vi "FPGA PID control.vi"(4 "PID output channel":T1, 5 "output ranges":T9={"output high (Inf)"=inf, "output low (-Inf)"=-inf}, 6 "reset pid":T7, 7 "PID gains":T8 {"filter coefficient" min=0 max=1; "proportional gain" step=0.125}, 8 "PID input channel":T1, 9 "setpoint":T5, 10 "set output":T3=[0.0, 0.0, 0.0, 0.0], 11 "inputs":T4=[0.0, 0.0, 0.0, 0.0]) -> (1 "PID status":T6, 2 "to AO channels":T2, 3 "actual outputs":sgl[](array[numeric]))   [LabVIEW 2016]
uses:
  Type Def Ctrls/FPGA ctrls/PID output selection.ctl
  <vilib>/rvi/Analysis/control/PID/Typedef/niFpgaPID_OutputRange.ctl
  <vilib>/rvi/Analysis/control/PID/Typedef/niFpgaPID_PIDGains.ctl
  Type Def Ctrls/FPGA ctrls/Reset PID.ctl
  Type Def Ctrls/FPGA ctrls/PID status.ctl
  Type Def Ctrls/FPGA ctrls/Manual Setpoint.ctl
  Type Def Ctrls/FPGA ctrls/Input Channels.ctl
  Type Def Ctrls/FPGA ctrls/Output Channels.ctl
  Type Def Ctrls/FPGA ctrls/AO channel cluster.ctl
  <vilib>/rvi/Emulation/niFpgaSctlEmulationGetInTimedLoop.vi
  <vilib>/rvi/Emulation/niFpgaProcessEmulError.vi
  <vilib>/rvi/Analysis/control/PID/SubVIs/niFpgaPID_PIDWrapper.vi
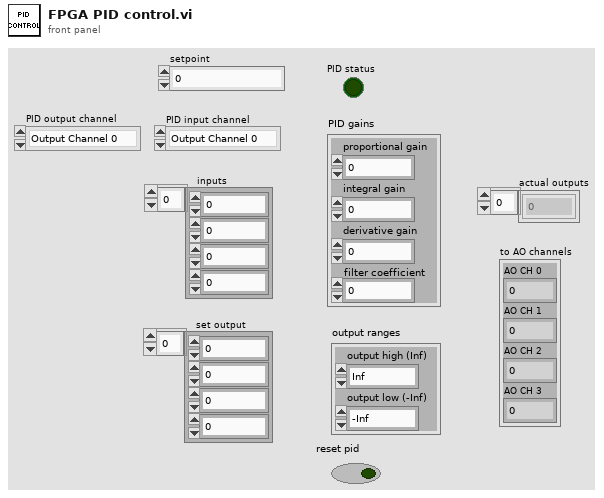
[diagram p1: front panel]
types:
  T1 = typedef "PID output selection.ctl" = enum16{"Output Channel 0", "Output Channel 1", "Output Channel 2", "Output Channel 3", "PID Disabled"}
  T2 = typedef "AO channel cluster.ctl" = cluster{"AO CH 0":fxp<+/-,20,5>, "AO CH 1":fxp<+/-,20,5>, "AO CH 2":fxp<+/-,20,5>, "AO CH 3":fxp<+/-,20,5>}
  T3 = typedef "Output Channels.ctl" = sgl[]
  T4 = typedef "Input Channels.ctl" = sgl[]
  T5 = typedef "Manual Setpoint.ctl" = sgl
  T6 = typedef "PID status.ctl" = bool
  T7 = typedef "Reset PID.ctl" = bool
  T8 = typedef "niFpgaPID_PIDGains.ctl" = cluster{"proportional gain":sgl, "integral gain":sgl, "derivative gain":sgl, "filter coefficient":sgl}
  T9 = typedef "niFpgaPID_OutputRange.ctl" = cluster{"output high (Inf)":sgl, "output low (-Inf)":sgl}
  T10 = cluster{"[0]":fxp<+/-,20,5>, "[1]":fxp<+/-,20,5>, "[2]":fxp<+/-,20,5>, "[3]":fxp<+/-,20,5>}
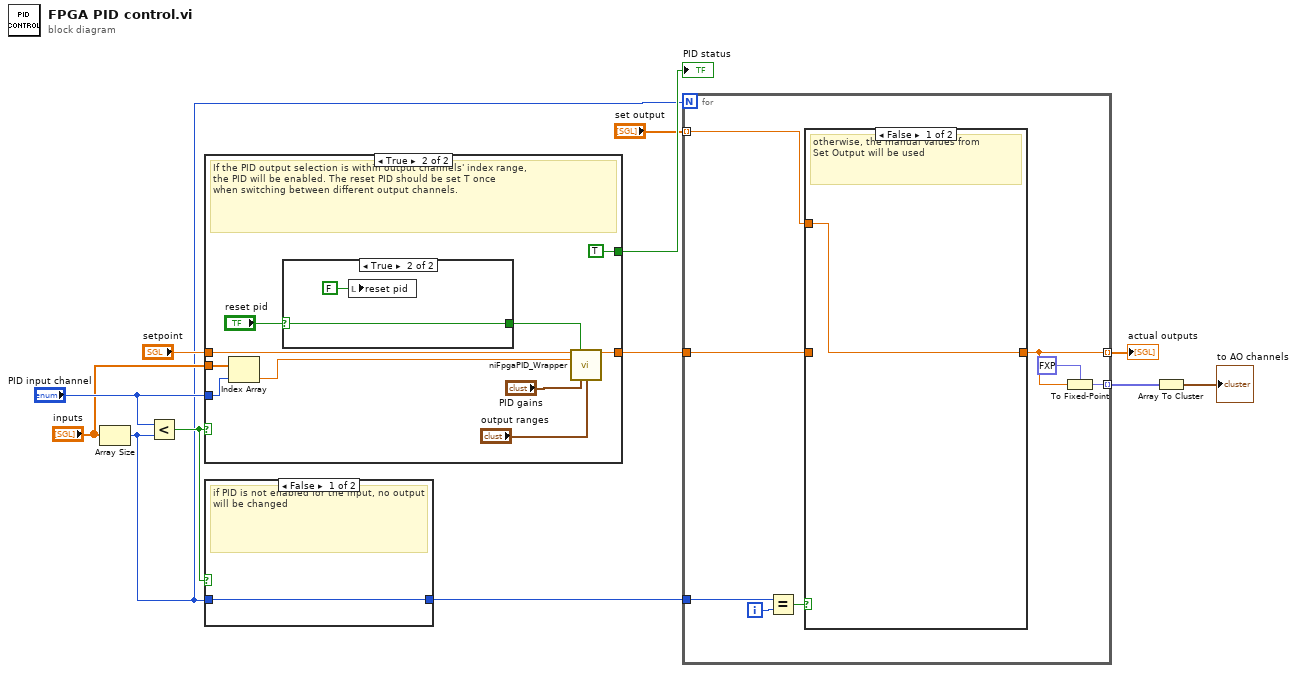
[diagram p0: block diagram]
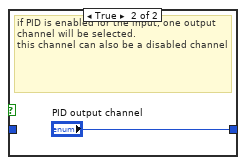
[diagram p2: hidden frame]
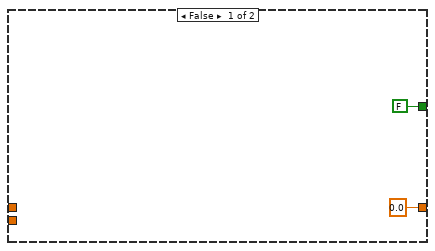
[diagram p4: hidden frame]
diagram:
  n1 = Array Size(array="inputs") -> (size(s)=w1:i32)
  n2 = Less?(x="PID input channel", y=w1) -> (x < y?=w2:bool)
  n3 = case shown="True" w2 {
    tunnel: "setpoint" -> [_ w24]
    tunnel: "PID input channel" -> [_ w22]
    tunnel: [sgl 0.0 ("output") w21] -> w11
    tunnel: "inputs" -> [_ w20]
    tunnel: [FALSE ("PID status") TRUE ("PID status")] -> w8
    frame False {
    }
    frame True {
      # "If the PID output selection is within output channels' index range,\nthe PID will be enabled. The reset PID should be set T once \nwhen switching between different output channels."
      n4 = Index Array(array=w20, index=w22) -> (element=w23:sgl)
      n5 = case shown="True" "reset pid" {
        selector: "reset pid" -> [w25 w27]
        tunnel: [w25 w27] -> w15
        frame False {
        }
        frame True {
          n6 = local write "reset pid"(T7 FALSE ("reset PID1?")) -> ()
        }
      }
      n7 = call-poly <vilib>:"niFpgaPID_Wrapper.vi"("setpoint"=w24, "reset? (F)"=w15, "process variable"=w23, "gains"="PID gains", "output range"="output ranges") -> ("output"=w21:sgl)  [unwired: 8 in, 2 out]
    }
  }
  "PID status" <- w8
  n8 = case shown="False" w2 {
    tunnel: [w28 "PID output channel"] -> w3
    tunnel: w1 -> [w28 _]
    frame False {
      # "if PID is not enabled for the input, no output will be changed"
    }
    frame True {
      # "if PID is enabled for the input, one output channel will be selected.\nthis channel can also be a disabled channel"
    }
  }
  n9 = for {
    N: w1 -> [_]
    tunnel: "set output" -> [w35] mode=indexing
    tunnel: w3 -> [w34]
    tunnel: w11 -> [w36]
    tunnel: [w31] -> w9 mode=indexing
    tunnel: [w30] -> w5 mode=indexing
    i -> [w32]
    n10 = Equal?(x=w34, y=w32) -> (x = y?=w37:bool)
    n11 = case shown="False" w37 {
      tunnel: [w38 w39] -> w31
      tunnel: w35 -> [w38 _]
      tunnel: w36 -> [_ w39]
      frame False {
        # "otherwise, the manual values from \nSet Output will be used"
      }
      frame True {
        # "when the index is the same as PID control channel, \nthe output from the PID will be used"
      }
    }
    n12 = To Fixed-Point(fixed-point type=fxp<+/-,20,5> 0.0 ("Mod1/AO0"), number=w31) -> (fixed-point=w30:fxp<+/-,20,5>)
  }
  "actual outputs" <- w9
  n13 = Array To Cluster(array=w5) -> (cluster=→"to AO channels":T10)
